vi "Camera.Simulated.SetBufferDependency.vi"(8 "error in (no error)":errorcluster, 10 "CircularBuffer.ImageData":refnum<class "CircularBuffer.ImageData.lvclass">, 11 "Camera.Simulated":refnum<class "Camera.Simulated.lvclass">) -> (0 "error out":errorcluster, 3 "Camera.Simulated":refnum<class "Camera.Simulated.lvclass">)   [LabVIEW 2013, in "Camera.Simulated.lvclass"]
doc: "---------------------------------------------------------------\nJKI State Machine Objects™\nhttp://jki.net/state-machine-objects/\nCopyright (C) 2005-2015, JKI <info@jki.net>\nALL RIGHTS RESERVEDJKI State Machine Objects (SMO) 1.0.0.4\nJKI - JKI\nCopyright (c) 2015, JKI"
uses:
  Camera.Simulated.lvclass
  CircularBuffer.ImageData/CircularBuffer.ImageData.lvclass
panel:
  # "For instructions on how to use the JKI State Machine Objects, examples and video tutorials, visit:\nhttp://jki.net/state-machine-objects/\n\nJKI State Machine Objects™\nhttp://jki.net/state-machine-objects/\nCopyright (C) 2005-2015, JKI <info@jki.net>\nALL RIGHTS RESERVED"
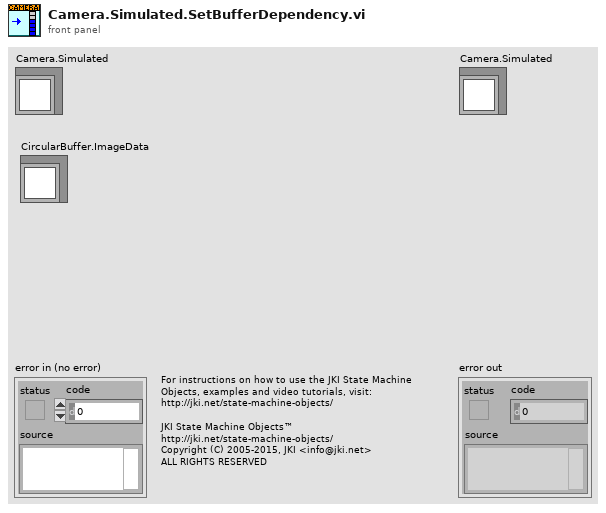
[diagram p1: front panel]
types:
  T1 = typedef "Camera.Simulated.lvclass/PrivateData--Ref.ctl" = refnum<data-value>
  T2 = typedef "Camera.Simulated.lvclass/PrivateData--Cluster.ctl" = cluster{"Dependencies":T3, "Configuration":T4}
  T3 = typedef "Camera.Simulated.lvclass/Dependencies--Cluster.ctl" = cluster{"CircularBuffer.ImageData":refnum<class "CircularBuffer.ImageData.lvclass">}
  T4 = typedef "Camera.Simulated.lvclass/Configuration--CLuster.ctl" = cluster{"Simulated Images Folder":path, "filetype":string}
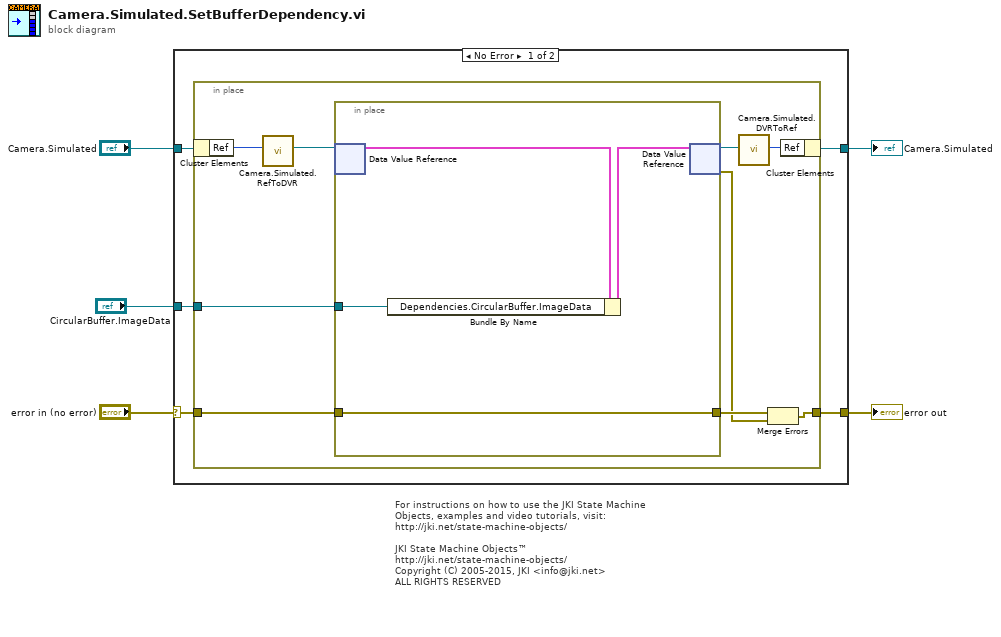
[diagram p0: block diagram]
diagram:
  # "For instructions on how to use the JKI State Machine Objects, examples and video tutorials, visit:\nhttp://jki.net/state-machine-objects/\n\nJKI State Machine Objects™\nhttp://jki.net/state-machine-objects/\nCopyright (C) 2005-2015, JKI <info@jki.net>\nALL RIGHTS RESERVED"
  n1 = case shown="No Error" "error in (no error)" {
    selector: "error in (no error)" -> [w8 w25]
    tunnel: [w7 w25] -> w4
    tunnel: [w9 w24] -> w5
    tunnel: "Camera.Simulated" -> [w10 w24]
    tunnel: "CircularBuffer.ImageData" -> [w6 _]
    frame No Error {
      n2 = in-place {
        in-place-border: w8 -> [w19]
        in-place-border: [w16] -> w7
        in-place-border: w6 -> [w15]
        n3 = in-place-cluster #1(w10) -> ("Ref"=w12:u32)
        n4 = call "Camera.Simulated.RefToDVR.vi"("Ref"=w12) -> ("Ref"=w11:T1)  [unwired: 10 in]
        n5 = in-place {
          in-place-border: w19 -> [w21]
          in-place-border: [w21] -> w18
          in-place-border: w15 -> [w20]
          n6 = in-place-dvr #2(w11) -> (w23:T2)  [unwired: 1 out]
          n7 = Bundle By Name(cluster=w23, "Dependencies.CircularBuffer.ImageData"=w20) -> (w22:T2)
          n8 = in-place-dvr #2(w22) -> (w14:T1, w17:errorcluster)
        }
        n9 = call "Camera.Simulated.DVRToRef.vi"("Ref"=w14) -> ("Ref"=w13:u32)  [unwired: 10 in]
        n10 = Merge Errors(w18, w17) -> (w16:errorcluster)
        n11 = in-place-cluster #1("Ref"=w13) -> (w9:refnum<class "Camera.Simulated.lvclass">)
      }
    }
    frame Error {
    }
  }
  "error out" <- w4
  "Camera.Simulated" <- w5
